vi "testerfile.vi"() -> ()   [LabVIEW 2015]
panel:
  out "Gauge":dbl(knob) scale=0.0..15.0
  in  "Slide":dbl(slide) scale=0.0..5.0
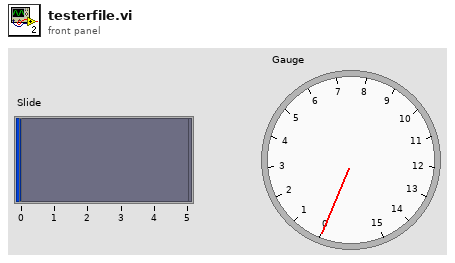
[diagram p1: front panel]
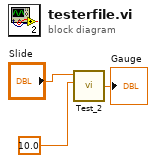
[diagram p0: block diagram]
diagram:
  n1 = call "Test_2.vi"("y"=10.0, "Slide"="Slide") -> ("Gauge"=→"Gauge":dbl)  [unwired: 9 in]
